vi "Sort into time.vi"(11 "Note Events in":T1[](array[typedef])) -> (3 "Note Events out":T1[](array[typedef]))   [LabVIEW 2016]
uses:
  Notes.ctl
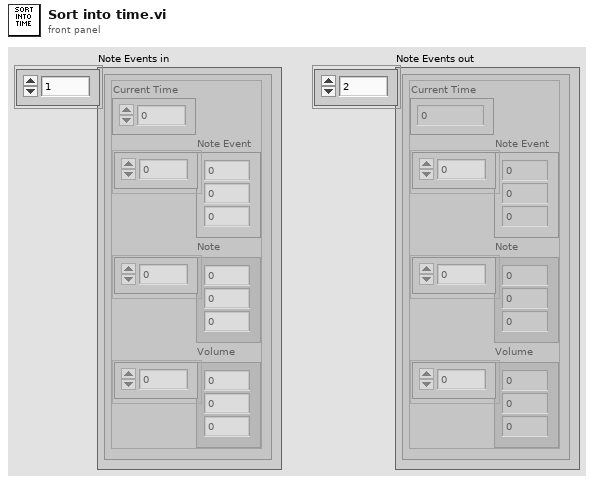
[diagram p1: front panel]
types:
  T1 = typedef "Notes.ctl" = cluster{"Current Time":u32, "Note Event":u32[], "Note":u32[], "Volume":u32[]}
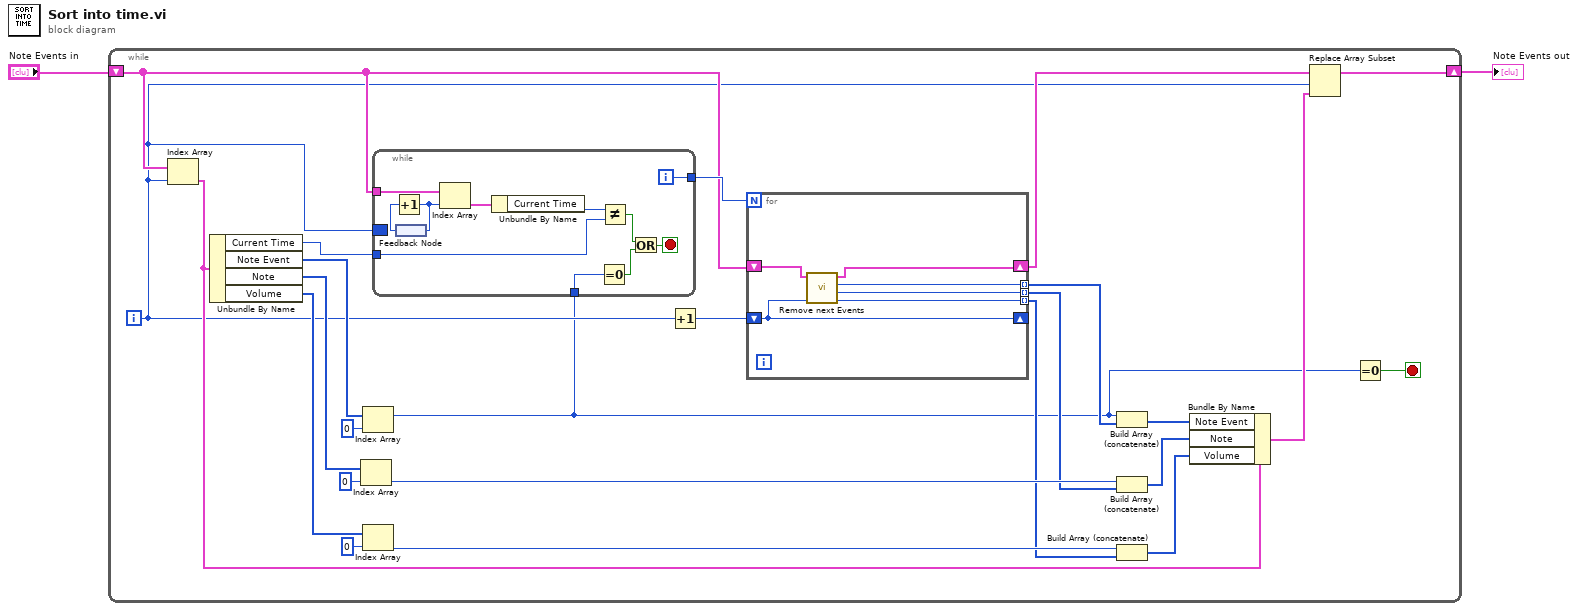
[diagram p0: block diagram]
diagram:
  n1 = while {
    shift-right: [w6] -> w1
    shift-left: "Note Events in" -> [w13]
    i -> [w5]
    stop <- w4 stop-if-true
    n2 = Index Array(array=w13, index=w5) -> (element=w9:T1)
    n3 = Unbundle By Name(w9) -> ("Current Time"=w27:u32, "Note Event"=w24:u32[], "Note"=w19:u32[], "Volume"=w18:u32[])
    n4 = Index Array(array=w19, index=0) -> (element=w17:u32)
    n5 = Index Array(array=w24, index=0) -> (element=w3:u32)
    n6 = Index Array(array=w18, index=0) -> (element=w16:u32)
    n7 = while {
      tunnel: w27 -> [w41]
      tunnel: w13 -> [w44]
      tunnel: [w40] -> w26
      border: w5 -> [_]
      tunnel: w3 -> [w34]
      i -> [w40]
      stop <- w36 stop-if-true
      n8 = feedback #1() -> (w38:i32)
      n9 = Increment(x=w38) -> (x+1=w39:i32)
      n10 = feedback-in #1(w39) -> ()
      n11 = Index Array(array=w44, index=w39) -> (element=w43:T1)
      n12 = Unbundle By Name(w43) -> ("Current Time"=w42:u32)
      n13 = Equal To 0?(x=w34) -> (x = 0?=w35:bool)
      n14 = Not Equal?(x=w42, y=w41) -> (x != y?=w37:bool)
      n15 = Or(x=w37, y=w35) -> (x .or. y?=w36:bool)
    }
    n16 = Increment(x=w5) -> (x+1=w25:i32)
    n17 = for {
      N: w26 -> [_]
      shift-right: [w29] -> w8
      shift-left: w13 -> [w28]
      shift-right: [w33] -> _
      shift-left: w25 -> [w33]
      tunnel: [w32] -> w14 mode=indexing
      tunnel: [w31] -> w15 mode=indexing
      tunnel: [w30] -> w23 mode=indexing
      n18 = call "Remove next Events.vi"("Note Events in"=w28, "Event Index"=w33) -> ("Note Events w/ subset deleted"=w29:T1[], "Note Event Removed"=w30:u32, "Note Removed"=w31:u32, "Volume Removed"=w32:u32)  [unwired: 5 in]
    }
    n19 = Build Array (concatenate)(w3, w23) -> (w12:u32[])
    n20 = Build Array (concatenate)(w17, w15) -> (w11:u32[])
    n21 = Build Array (concatenate)(w16, w14) -> (w10:u32[])
    n22 = Bundle By Name(cluster=w9, "Note Event"=w12, "Note"=w11, "Volume"=w10) -> (w7:T1)
    n23 = Replace Array Subset(array=w8, new element=w7, index=w5) -> (w6:T1[])
    n24 = Equal To 0?(x=w3) -> (x = 0?=w4:bool)
  }
  "Note Events out" <- w1
